vi "Main.vi"(8 "error in (no error)":errorcluster, 11 "Example Class A in":refnum<class "ExampleClassA.lvclass">) -> (0 "error out":errorcluster, 3 "Example Class A out":refnum<class "ExampleClassA.lvclass">)   [LabVIEW 2012, in "ExampleClassA.lvclass"]
doc: "Main VI and GUI of this example component."
uses:
  ExampleClassA.lvclass
  <vilib>/Distrio/Murmex/InitialiseMessage/InitialiseMessage.lvclass
  <vilib>/Distrio/Murmex/Murmex/data_compression_enum.ctl
  ExampleClassA.lvclass/ExampleClassA.ctl
  <vilib>/Distrio/Murmex/ConfigureMessage/ConfigureMessage.lvclass
  <vilib>/Distrio/Murmex/StopMessage/StopMessage.lvclass
  <vilib>/Distrio/Murmex/StartMessage/StartMessage.lvclass
  <vilib>/Distrio/Murmex/StartMessage/run mode enum.ctl
  <vilib>/Distrio/Murmex/Murmex/update_cluster.ctl
  <vilib>/Distrio/Murmex/TerminateMessage/TerminateMessage.lvclass
  <vilib>/Distrio/Murmex/Murmex/Set configure at initialise.vi
  <vilib>/Distrio/Murmex/Murmex/Set VI reference.vi
  <vilib>/Distrio/Murmex/Murmex/Get ID.vi
  <vilib>/Distrio/Murmex/Murmex/Set log reference.vi
  <vilib>/Distrio/Murmex/Murmex/Set data compression.vi
  <vilib>/Distrio/Murmex/StartMessage/Set run mode.vi
  <vilib>/Distrio/Murmex/Murmex/Murmex.lvclass
panel:
  out "log":string
  in  "Tab Control":enum32{"User", "Debug"}(tab)
  in  "number of channels":i32=2
  in  "button:configure":bool
  in  "data blocks to generate":i32=5
  in  "period":dbl[unit]=0.5
  in  "button:send_data?":bool
  in  "button:quit":bool
  in  "component ID":string
  out "terminated?":bool
  out "main loop counter":i32
  out "component A":refnum<class "ExampleClassA.lvclass">
  # "IMPORTANT: When starting this VI directly, enter its ID on the Debug tab."
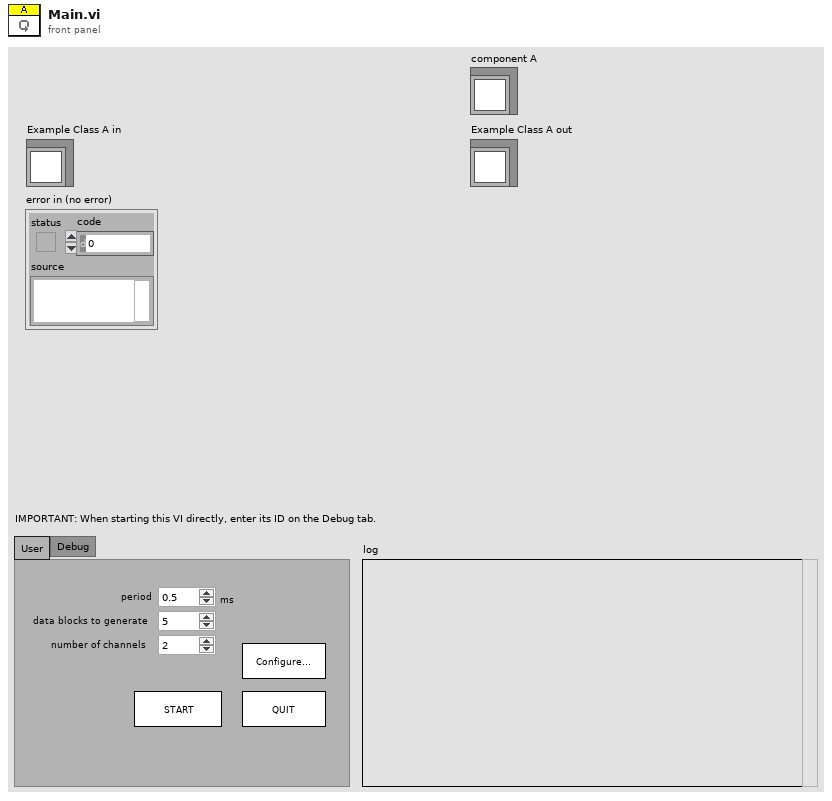
[diagram p1: front panel]
types:
  T1 = typedef "Murmex.lvlib/Murmex.lvclass/data_compression_enum.ctl" = enum16{"base64", "zip+base64", "byte to string"}
  T2 = typedef "Murmex.lvlib/StartMessage.lvclass/run mode enum.ctl" = enum16{"infinite", "finite"}
  T3 = typedef "Murmex.lvlib/Murmex.lvclass/update_cluster.ctl" = cluster{"target ID":string, "key chains":string[], "values":variant[]}
  T4 = enum8{"Enabled", "Disabled", "Disabled and Grayed Out"}
  T5 = typedef "Murmex.lvclass/command_enum.ctl" = enum16{"null", "initialise", "reset", "terminate", "acknowledge", "update", "inspect", "inform", "proceed", "start", "stop", "fetch", "configure", "generic"}
  T6 = typedef "Murmex.lvclass/Event type enumerations.ctl" = enum16{"before", "after"}
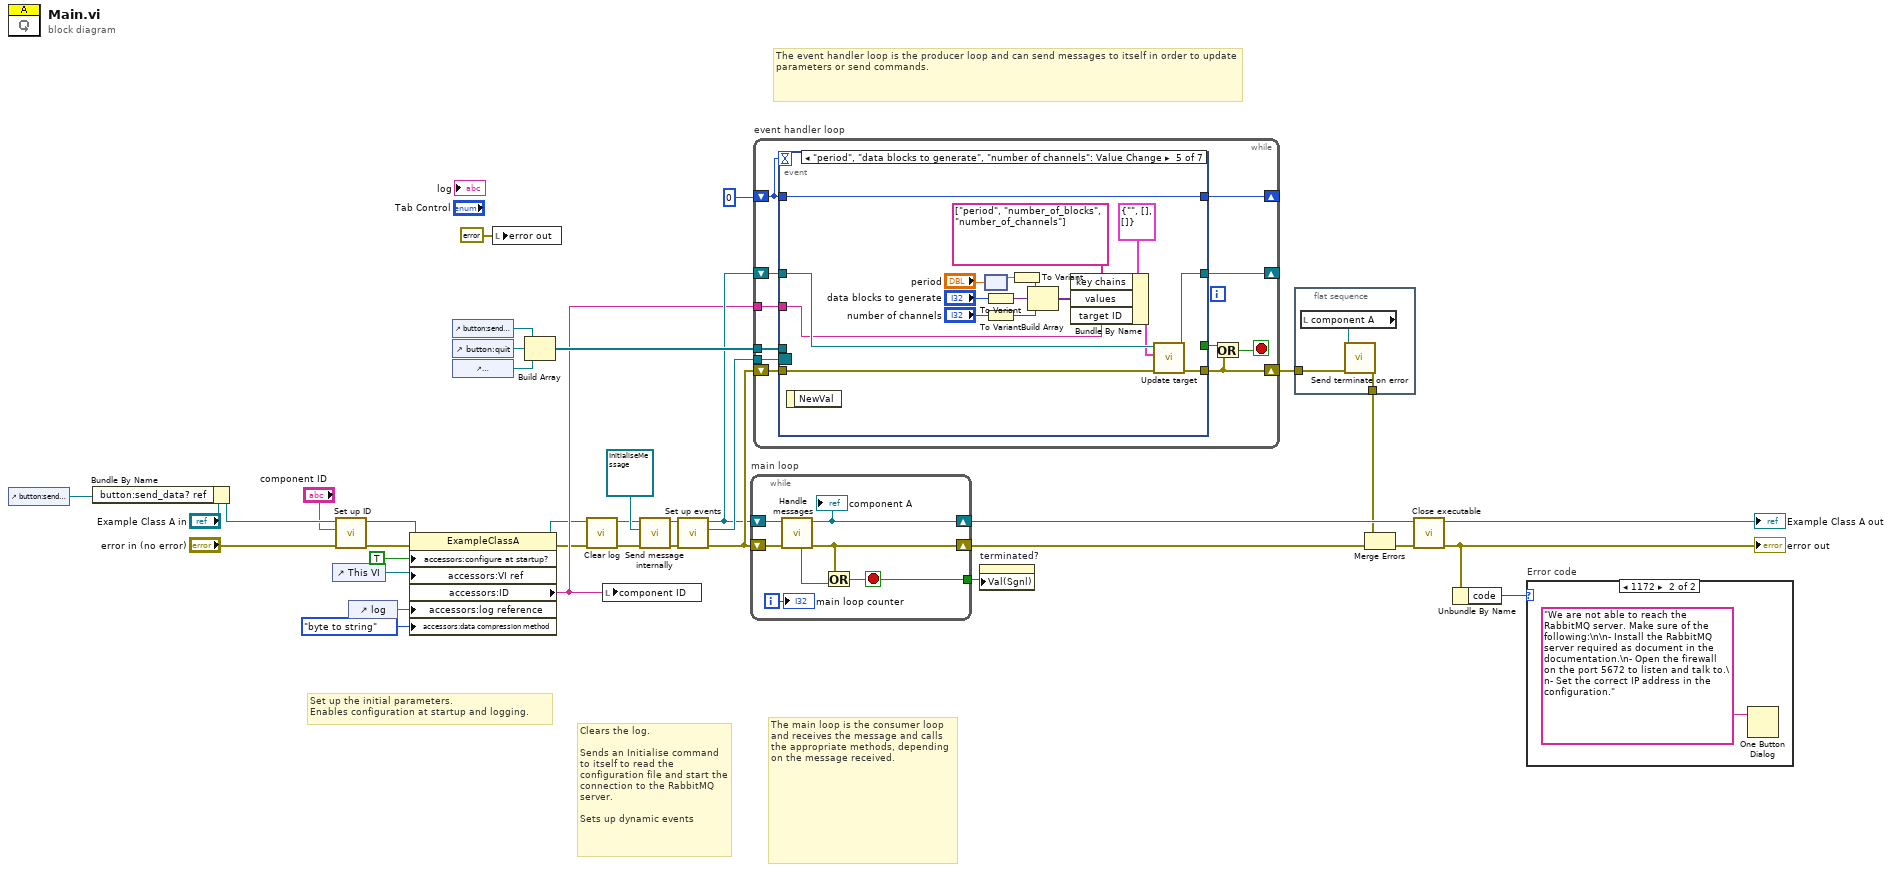
[diagram p0: block diagram]
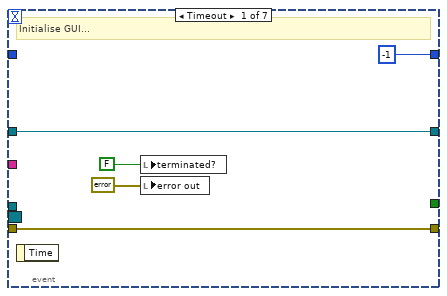
[diagram p3: hidden frame]
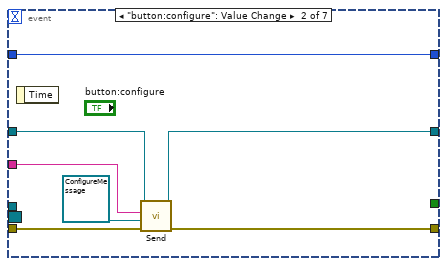
[diagram p4: hidden frame]
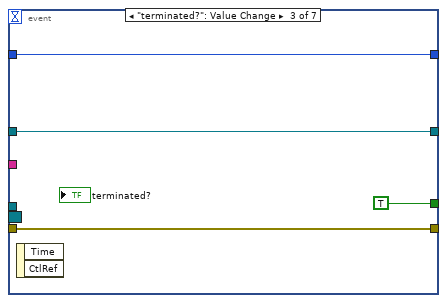
[diagram p5: hidden frame]
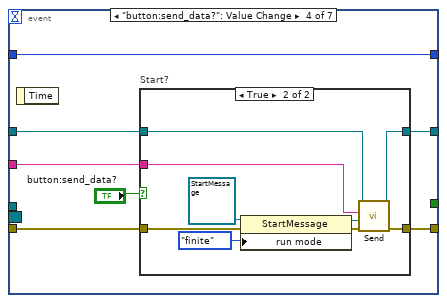
[diagram p6: hidden frame]
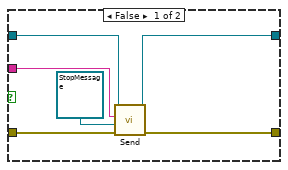
[diagram p7: hidden frame]
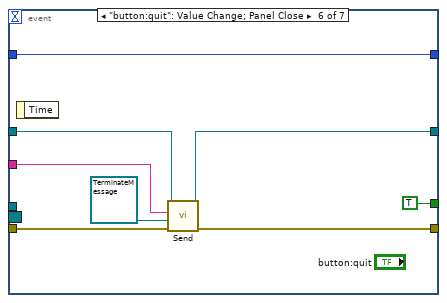
[diagram p8: hidden frame]
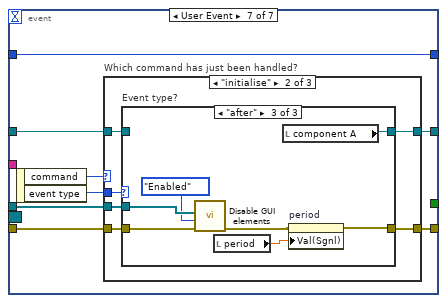
[diagram p9: hidden frame]
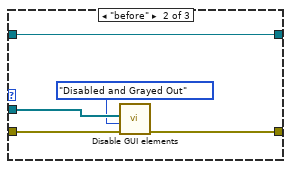
[diagram p12: hidden frame]
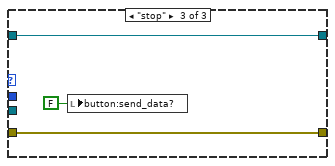
[diagram p13: hidden frame]
diagram:
  # "The event handler loop is the producer loop and can send messages to itself in order to update parameters or send commands."
  # "The main loop is the consumer loop and receives the message and calls the appropriate methods, depending on the message received."
  # "Clears the log.\n\nSends an Initialise command to itself to read the configuration file and start the connection to the RabbitMQ server.\n\nSets up dynamic events"
  # "Set up the initial parameters. \nEnables configuration at startup and logging."
  n1 = control-ref of="button:send_data?"() -> (w33:refnum<vi>)
  n2 = Bundle By Name(cluster="Example Class A in", "button:send_data? ref"=w33) -> (w34:refnum<class "ExampleClassA.lvclass">)
  n3 = control-ref of="This VI"() -> (w13:refnum<vi>)
  n4 = call <vilib>:"Set up ID.vi"("error in (no error)"="error in (no error)", "component ID"="component ID", "MurmexBase in"=w34) -> ("error out"=w11:errorcluster, "MurmexBase out"=w10:refnum<class "ExampleClassA.lvclass">)  [unwired: 6 in, 1 out]
  n5 = control-ref of="log"() -> (w8:refnum<vi>)
  n6 = property class="ExampleClassA"(reference=w10, error in=w11, "accessors:configure at startup?"=TRUE ("configure at startup?"), "accessors:VI ref"=w13, "accessors:log reference"=w8, "accessors:data compression method"=data_compression_enum."byte to string" ("data compression method")) -> (reference out=w5:refnum<class "ExampleClassA.lvclass">, error out=w7:errorcluster, "accessors:ID"=w9:string)
  n7 = control-ref of="button:send_data?"() -> (w22:refnum<vi>)
  n8 = control-ref of="button:quit"() -> (w23:refnum<vi>)
  n9 = control-ref of="button:configure"() -> (w20:refnum<vi>)
  n10 = local write "error out"(errorcluster {"status"=FALSE, "code"=0, "source"=""} ("error out")) -> ()
  n11 = Build Array(w22, w23, w20) -> (w21:refnum<vi>[])
  n12 = call <vilib>:"Clear log.vi"("error in (no error)"=w7, "MurmexBase in"=w5) -> ("error out"=w6:errorcluster, "MurmexBase out"=w4:refnum<class "ExampleClassA.lvclass">)  [unwired: 8 in]
  n13 = local write "component ID"(w9) -> ()
  n14 = call <vilib>:"Send message internally.vi"("error in (no error)"=w6, "Message"=refnum<class "InitialiseMessage.lvclass"> refnum ("InitialiseMessage.lvclass"), "Murmex in"=w4) -> ("error out"=w27:errorcluster, "Murmex out"=w26:refnum<class "ExampleClassA.lvclass">)  [unwired: 7 in]
  n15 = call <vilib>:"Set up events.vi"("error in (no error)"=w27, "MurmexBase in"=w26) -> ("error out"=w24:errorcluster, "Event Registration Refnum"=w25:refnum<event-registration>, "MurmexBase out"=w14:refnum<class "ExampleClassA.lvclass">)  [unwired: 7 in]
  n16 = while "main loop" {
    tunnel: [w39] -> w28
    shift-right: [w40] -> w32
    shift-left: w24 -> [w43]
    shift-right: [w44] -> w18
    shift-left: w14 -> [w42]
    i -> [w38]
    stop <- w39 stop-if-true
    n17 = call <vilib>:"Handle messages.vi"("error in (no error)"=w43, "Murmex in"=w42) -> ("error out"=w40:errorcluster, "Murmex out"=w44:refnum<class "ExampleClassA.lvclass">, "terminated?"=w41:bool)  [unwired: 7 in]
    "component A" <- w44
    n18 = Or(x=w40, y=w41) -> (x .or. y?=w39:bool)
    "main loop counter" <- w38
  }
  n19 = while "event handler loop" {
    shift-right: [w53] -> _
    shift-left: 0 -> [w54]
    shift-right: [w49] -> w17
    shift-left: w24 -> [w55]
    tunnel: w25 -> [w52]
    tunnel: w21 -> [w51]
    tunnel: w9 -> [w47]
    shift-right: [w45] -> _
    shift-left: w14 -> [w46]
    stop <- w48 stop-if-true
    n20 = event shown="[4] \"period\", \"data blocks to generate\", \"number of channels\": Value Change" {
      selector: w52 -> [_ _ _ _ _ _ _]
      dyn-events: _ -> [_ _ _ _ _ _ _]
      timeout: w54 -> [_ _ _ _ _ _ _]
      tunnel: [_ _ TRUE _ _ TRUE _] -> w50
      tunnel: [w57 w65 w71 w77 w94 w112 w123] -> w49
      tunnel: w55 -> [w57 w66 w71 w76 w107 w113 w124]
      tunnel: [-1 w67 w70 w78 w109 w116 w125] -> w53
      tunnel: w54 -> [_ w67 w70 w78 w109 w116 w125]
      tunnel: w51 -> [_ _ _ _ _ _ w121]
      tunnel: w47 -> [_ w64 _ w74 w102 w115 _]
      tunnel: w46 -> [w56 w62 w68 w73 w103 w111 w119]
      tunnel: [w56 w61 w68 w72 w95 w110 w118] -> w45
      event Timeout {
        # "Initialise GUI..."
        n21 = event-data() -> ()  [unwired: 1 in, 1 out]
        n22 = local write "terminated?"(FALSE ("terminated?")) -> ()
        n23 = local write "error out"(errorcluster {"status"=FALSE, "code"=0, "source"=""} ("error out")) -> ()
      }
      event "button:configure": Value Change {
        n24 = event-data() -> ()  [unwired: 1 in, 1 out]
        n25 = call <vilib>:"Send.vi"("error in (no error)"=w66, "Message"=refnum<class "ConfigureMessage.lvclass"> refnum ("ConfigureMessage.lvclass"), "recipient"=w64, "Murmex in"=w62) -> ("error out"=w65:errorcluster, "Murmex out"=w61:refnum<class "ExampleClassA.lvclass">)  [unwired: 6 in]
      }
      event "terminated?": Value Change {
        n26 = event-data() -> ()  [unwired: 1 in, 2 out]
      }
      event "button:send_data?": Value Change {
        n27 = event-data() -> ()  [unwired: 1 in, 1 out]
        n28 = case "Start?" shown="True" "button:send_data?" {
          tunnel: [w83 w92] -> w77
          tunnel: w76 -> [w84 w89]
          tunnel: w74 -> [w81 w85]
          tunnel: w73 -> [w79 w91]
          tunnel: [w80 w90] -> w72
          frame False {
            n29 = call <vilib>:"Send.vi"("error in (no error)"=w84, "Message"=refnum<class "StopMessage.lvclass"> refnum ("StopMessage.lvclass"), "recipient"=w81, "Murmex in"=w79) -> ("error out"=w83:errorcluster, "Murmex out"=w80:refnum<class "ExampleClassA.lvclass">)  [unwired: 6 in]
          }
          frame True {
            n30 = property class="StartMessage"(reference=refnum<class "StartMessage.lvclass"> refnum ("StartMessage.lvclass"), error in=w89, "run mode"=run_mode_enum."finite") -> (reference out=w87:refnum<class "StartMessage.lvclass">)  [unwired: 1 out]
            n31 = call <vilib>:"Send.vi"("error in (no error)"=w89, "Message"=w87, "recipient"=w85, "Murmex in"=w91) -> ("error out"=w92:errorcluster, "Murmex out"=w90:refnum<class "ExampleClassA.lvclass">)  [unwired: 6 in]
          }
        }
      }
      event "period", "data blocks to generate", "number of channels": Value Change {
        n32 = event-data() -> ()  [unwired: 1 in, 1 out]
        n33 = node("period") -> (w96:dbl)
        n34 = To Variant(anything="data blocks to generate") -> (Variant=w101:variant)
        n35 = To Variant(anything="number of channels") -> (Variant=w98:variant)
        n36 = To Variant(anything=w96) -> (Variant=w97:variant)
        n37 = Build Array(w97, w101, w98) -> (w104:variant[])
        n38 = Bundle By Name(cluster=T3 {"target ID"="", "key chains"=[], "values"=[]} ("update cluster"), "key chains"=string[] ["period", "number_of_blocks", "number_of_channels"], "values"=w104, "target ID"=w102) -> (w93:T3)
        n39 = call <vilib>:"Update target.vi"("error in (no error)"=w107, "update cluster"=w93, "MurmexBase in"=w103) -> ("error out"=w94:errorcluster, "MurmexBase out"=w95:refnum<class "ExampleClassA.lvclass">)  [unwired: 7 in]
      }
      event "button:quit": Value Change; Panel Close {
        n40 = event-data() -> ()  [unwired: 1 in, 1 out]
        n41 = call <vilib>:"Send.vi"("error in (no error)"=w113, "Message"=refnum<class "TerminateMessage.lvclass"> refnum ("TerminateMessage.lvclass"), "recipient"=w115, "Murmex in"=w111) -> ("error out"=w112:errorcluster, "Murmex out"=w110:refnum<class "ExampleClassA.lvclass">)  [unwired: 6 in]
      }
      event User Event {
        n42 = event-data() -> ("command"=w122:T5, "event type"=w120:T6)  [unwired: 1 in]
        n43 = case "Which command has just been handled?" shown="\"initialise\"" w122 {
          tunnel: w124 -> [w127 w133 w150]
          tunnel: [w127 w130 w150] -> w123
          tunnel: w121 -> [_ w132 _]
          tunnel: w120 -> [_ w131 _]
          tunnel: w119 -> [w126 w129 w148]
          tunnel: [w126 w128 w148] -> w118
          frame Default {
          }
          frame "initialise" {
            n44 = case "Event type?" shown="\"after\"" w131 {
              tunnel: w133 -> [w135 w140 w145]
              tunnel: w132 -> [_ w138 w147]
              tunnel: [w135 w139 w142] -> w130
              tunnel: w129 -> [w134 w136 _]
              tunnel: [w134 w136 w141] -> w128
              frame Default {
              }
              frame "before" {
                n45 = call <vilib>:"Disable GUI elements.vi"("error in (no error)"=w140, "enabled state"=T4."Disabled and Grayed Out" ("Disabled"), "control refs"=w138) -> ("error out"=w139:errorcluster)  [unwired: 8 in]
              }
              frame "after" {
                n46 = call <vilib>:"Disable GUI elements.vi"("error in (no error)"=w145, "enabled state"=T4."Enabled" ("Disabled"), "control refs"=w147) -> ("error out"=w143:errorcluster)  [unwired: 8 in]
                n47 = local read "period"() -> (w144:dbl[unit])
                n48 = local read "component A"() -> (w141:refnum<class "ExampleClassA.lvclass">)
                n49 = property on="period" class="DigNum (strict)"(error in=w143, "Val(Sgnl)"=w144) -> (error out=w142:errorcluster)  [unwired: 1 in, 1 out]
              }
            }
          }
          frame "stop" {
            n50 = local write "button:send_data?"(FALSE ("button:send_data?")) -> ()
          }
        }
      }
    }
    n51 = Or(x=w50, y=w49) -> (x .or. y?=w48:bool)
  }
  n52 = property on="terminated?" class="Bool (strict)"("Val(Sgnl)"=w28) -> ()  [unwired: 2 in, 2 out]
  n53 = flat-sequence {
    tunnel: w17 -> [w153]
    tunnel: [w152] -> w16
    frame #0 {
      n54 = local read "component A"() -> (w151:refnum<class "ExampleClassA.lvclass">)
      n55 = call <vilib>:"Send terminate on error.vi"("error in (no error)"=w153, "Murmex in"=w151) -> ("error out"=w152:errorcluster)  [unwired: 8 in, 1 out]
    }
  }
  n56 = Merge Errors(w16, w32) -> (w19:errorcluster)
  n57 = call <vilib>:"Close executable.vi"("error in (no error)"=w19, "MurmexBase in"=w18) -> ("error out"=w2:errorcluster, "MurmexBase out"=→"Example Class A out":refnum<class "ExampleClassA.lvclass">)  [unwired: 8 in]
  "error out" <- w2
  n58 = Unbundle By Name(w2) -> ("code"=w1:i32)
  n59 = case "Error code" shown="1172" w1 {
    frame Default {
    }
    frame 1172 {
      n60 = One Button Dialog(message="We are not able to reach the RabbitMQ server. Make sure of the following:\n\n- Install the RabbitMQ server required as document in the documentation.\n- Open the firewall on the port 5672 to listen and talk to.\n- Set the correct IP address in the configuration.") -> ()  [unwired: 1 in, 1 out]
    }
  }
